vi "String Array to INI.vi"(0 "Path":path, 5 "Section":string, 9 "Array":string[][](array[string]), 11 "Error IN":errorcluster) -> (15 "Error OUT":errorcluster)   [LabVIEW 2013]
uses:
  <vilib>/Utility/config.llb/Write Key (String).vi
  <vilib>/Utility/config.llb/NI_LVConfig.lvlib
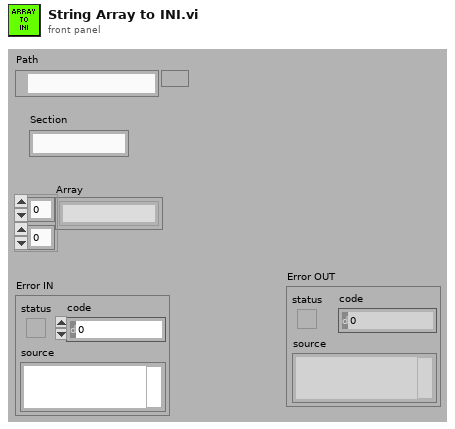
[diagram p1: front panel]
types:
  T1 = typedef "NI_LVConfig.lvlib/Config Data RefNum.ctl" = refnum<k1>
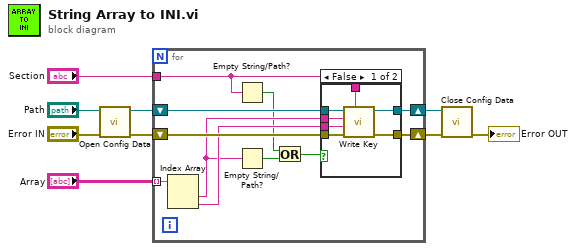
[diagram p0: block diagram]
diagram:
  n1 = call <vilib>:"Open Config Data.vi"("error in (no error)"="Error IN", "configuration file path"="Path") -> ("error out"=w6:errorcluster, "refnum"=w7:T1)  [unwired: 7 in, 1 out]
  n2 = for {
    tunnel: "Array" -> [w16] mode=indexing
    tunnel: "Section" -> [w13]
    shift-right: [w19] -> w3
    shift-left: w6 -> [w20]
    shift-right: [w18] -> w2
    shift-left: w7 -> [w17]
    n3 = Index Array(array=w16) -> (element #1=w14:string, element #2=w15:string)  [unwired: 2 in]
    n4 = Empty String/Path?(string/path=w13) -> (empty?=w11:bool)
    n5 = Empty String/Path?(string/path=w14) -> (empty?=w12:bool)
    n6 = Or(x=w11, y=w12) -> (x .or. y?=w10:bool)
    n7 = case shown="False" w10 {
      tunnel: w20 -> [w27 w28]
      tunnel: w13 -> [w26 _]
      tunnel: [w25 w28] -> w19
      tunnel: [w24 w29] -> w18
      tunnel: w17 -> [w23 w29]
      tunnel: w14 -> [w22 _]
      tunnel: w15 -> [w21 _]
      frame False {
        n8 = call-poly <vilib>:"Write Key.vi"("section"=w26, "error in (no error)"=w27, "value"=w21, "key"=w22, "refnum"=w23) -> ("error out"=w25:errorcluster, "refnum out"=w24:T1)  [unwired: 4 in, 1 out]
      }
      frame True {
      }
    }
  }
  n9 = call <vilib>:"Close Config Data.vi"("error in (no error)"=w3, "refnum"=w2) -> ("error out"=→"Error OUT":errorcluster)  [unwired: 8 in, 1 out]
